vi "Set Kasli Name from ID.vi"(8 "error in (no error)":errorcluster, 11 "Kasli Wrapper 2.0 in":refnum<class "Kasli Wrapper 2.0.lvclass">) -> (0 "error out":errorcluster, 2 "Kasli Name":string, 3 "Kasli Wrapper 2.0 out":refnum<class "Kasli Wrapper 2.0.lvclass">, 4 "Dummy?":bool)   [LabVIEW 2020, in "TALOS.lvlib" / "Kasli Wrapper 2.0.lvlib" / "Kasli Wrapper 2.0.lvclass"]
doc: "This VI interprets the Kasli Name based on the uService ID"
uses:
  Kasli Wrapper 2.0.lvclass
  C:/LabVIEW Code/TALOS/talos/Ancestor/Ancestor/Ancestor.lvclass
  Ancestor/Ancestor/Ancestor.lvclass/Ancestor.ctl
  Ancestor/Ancestor/Read ID.vi
  Support VIs/Generate Error.vi
  FGV/Error Memory/Get Error Description.vi
  Support VIs/Get PC name.vi
  Support VIs/Get Class Name.vi
  <vilib>/Utility/error.llb/Clear Errors.vi
  FGV/Error Memory/Error Memory Core.vi
  <vilib>/AdvancedString/Delimited String to 1D String Array.vi
  Support VIs/Circus Root Path.vi
  FGV/Error Memory/Error Crt Lvl checker.vi
  FGV/Error Memory/Error Memory Core.vi/40c8088d-b597-4017-91af-faa98e00292e.vi
  FGV/Error Memory/Error Memory Core.vi/d4a3ab98-063c-4e44-b43d-fbdcfe6c2be2.vi
  Support VIs/Global Memory.vi
  <vilib>/Utility/LVClass/Get LV Class Name.vi
  Support VIs/Is in Packed Library.vi
  Support VIs/TALOS Root path.vi
  Support VIs/Read CSV worksheet.vi
  Support VIs/Global Constants.vi
  <vilib>/Utility/error.llb/General Error Handler.vi
  Support VIs/Error Log.vi
  Ancestor/Ancestor/Ancestor.lvclass
  <vilib>/Comparison/Equal/Equal Functor/Equal Functor.lvclass
  TALOS.lvlib
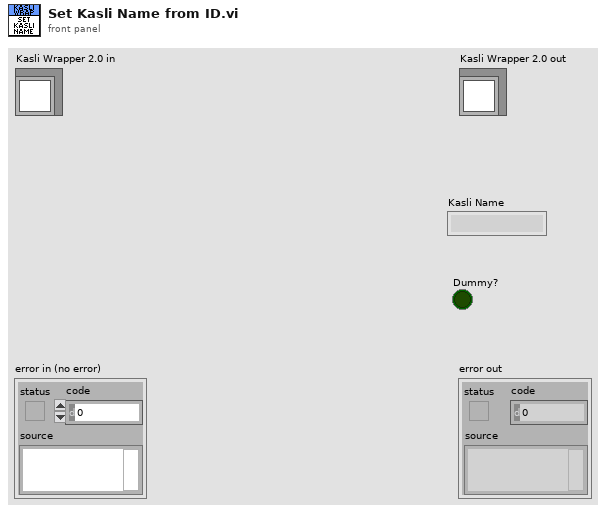
[diagram p1: front panel]
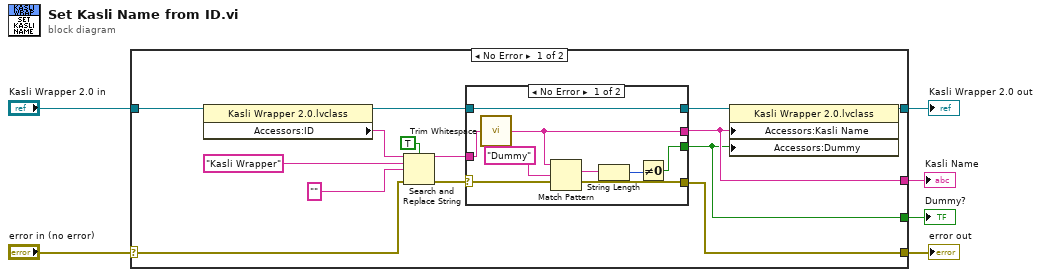
[diagram p0: block diagram]
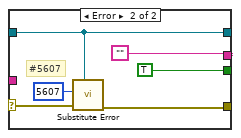
[diagram p2: hidden frame]
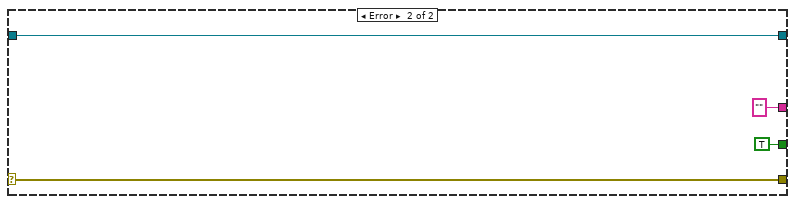
[diagram p3: hidden frame]
diagram:
  n1 = case shown="No Error" "error in (no error)" {
    selector: "error in (no error)" -> [w15 w38]
    tunnel: [w12 w38] -> w5
    tunnel: [w9 w37] -> w3
    tunnel: "Kasli Wrapper 2.0 in" -> [w20 w37]
    tunnel: [w8 "" ("trimmed string")] -> w2
    tunnel: [w7 TRUE ("Dummy")] -> w1
    frame No Error {
      n2 = property class="Kasli Wrapper 2.0.lvclass"(reference=w20) -> (reference out=w11:refnum<class "Kasli Wrapper 2.0.lvclass">, "Accessors:ID"=w19:string)  [unwired: 1 in, 1 out]
      n3 = Search and Replace String(case sensitive?=TRUE ("ignore case? (F)"), input string=w19, search string="Kasli Wrapper", replace string="" ("replace string (\"\")"), error in=w15) -> (result string=w13:string, error out=w14:errorcluster)  [unwired: 3 in, 2 out]
      n4 = case shown="No Error" w14 {
        selector: w14 -> [w27 w34]
        tunnel: w13 -> [w28 _]
        tunnel: [w27 w33] -> w12
        tunnel: [w23 TRUE ("Dummy")] -> w7
        tunnel: [w22 ""] -> w8
        tunnel: w11 -> [w21 w31]
        tunnel: [w21 w31] -> w10
        frame No Error {
          n5 = call <vilib>:"Trim Whitespace.vi"("string"=w28) -> ("trimmed string"=w22:string)  [unwired: 1 in]
          n6 = Match Pattern(string=w22, regular expression="Dummy") -> (match substring=w25:string)  [unwired: 1 in, 3 out]
          n7 = String Length(string=w25) -> (length=w24:i32)
          n8 = Not Equal To 0?(x=w24) -> (x != 0?=w23:bool)
        }
        frame Error {
          # "#5607"
          n9 = call "Substitute Error.vi"("LabVIEW Object"=w31, "error in (no error)"=w34, "Error Code"=5607) -> ("error out"=w33:errorcluster)  [unwired: 8 in]
        }
      }
      n10 = property class="Kasli Wrapper 2.0.lvclass"(reference=w10, "Accessors:Kasli Name"=w8, "Accessors:Dummy"=w7) -> (reference out=w9:refnum<class "Kasli Wrapper 2.0.lvclass">)  [unwired: 1 in, 1 out]
    }
    frame Error {
    }
  }
  "error out" <- w5
  "Kasli Wrapper 2.0 out" <- w3
  "Kasli Name" <- w2
  "Dummy?" <- w1
